vi "CODMn通讯.vi"() -> ()   [LabVIEW 2016, in "斯坦道CODMn新电路板.lvlib"]
uses:
  <vilib>/NI/Modbus Library/API/Wrapper/Create TCP Slave.vi
  <vilib>/Utility/config.llb/Write Key (String).vi
  <vilib>/Plasmionique/MB Master/MB_Master/MB_Master.lvclass
  <vilib>/NI/Modbus Library/API/Slave/Modbus Slave.lvclass
  <vilib>/Utility/config.llb/NI_LVConfig.lvlib
  <vilib>/Plasmionique/MB Master/MB Master.lvlib
  <vilib>/NI/Modbus Library/API/Wrapper/API Main.lvlib
panel:
  out "控制命令 2":u16[](array[numeric]) format="%xH"
  out "状态告警区":T1 {"工作状态" items=["空闲"=0, "水样测试"=1, "标样核查"=2, "零点核查"=3, "跨度核查"=4, "空白测试"=5, "平行样测试"=6, "加标回收"=7, "空白校准"=8, "标样校准"=9, "初始化（清洗）"=10, "调试"=22, "填充管路"=30, "清洗管路"=31, "清洗反应杯"=32]; "告警代码" items=["无告警", "缺试剂告警", "缺水样告警", "缺蒸馏水告警", "缺标液告警", "仪表漏液告警", "标定异常告警", "超量程告警", "加热异常", "低试剂预警", "超上限告警", "超下限告警", "仪表内部其他异常", "滴定异常告警", "电极异常告警", "量程切换告警", "参数设置告警", "PH电极电位异常", "电导率电极异常", "浊度光度异常", "溶解氧电极异常", "溶解氧光强异常", "温度异常告警", "PH异常告警", "溶解氧异常告警", "电导率异常告警", "浊度异常告警", "叶绿素异常告警", "藻密度异常告警", "蓝绿藻异常告警", "ORP异常告警", "氨氮异常告警", "清洁刷异常告警", "SD卡异常告警", "蓝牙异常告警", "Wifi异常告警", "流程异常告警"]; "故障代码" items=["无故障", "电机故障", "温度故障", "通讯故障", "滴定故障"]}
  out "测量数据区":T2 {"单位" items=["ug/L", "mg/L", "ppm", "mg/m3", "cm", "ppb", "ug/m3", "%", "nmol/mol", "umol/mol", "MPN/L", "MPN/100ml", "ng/m3", "NTU", "无量纲", "ms/cm", "us/cm", "℃", "mV", "万个/L"]}
  out "状态告警区":u16[](array[numeric])
  out "测量数据区":u16[](array[numeric])
  out "序列号":string
  out "status":bool
  out "关键参数区":T3
  in  "读关键参数区":bool
  in  "读状态告警区":bool
  in  "读测量数据区":bool
  in  "站号":u16(ring) items=["CODMn"=21, "氨氮"=3]
  in  "停止":bool
  in  "启动":bool
  in  "控制命令":u16(ring) items=["启动测量"=1, "标样核查"=2, "零点核查"=3, "跨度核查"=4, "空白测试"=5, "平行样测试"=6, "加标回收"=7, "空白校准"=8, "标样校准"=9, "初始化（清洗）"=10, "停止测试"=11, "仪器重启"=12, "校时"=13, "模式设置"=14, "测量间隔设置"=15]
  in  "控制命令参数":u16[](array[numeric]) format="%04xH"
  in  "VISA Resource":refnum<visa-resource-name>
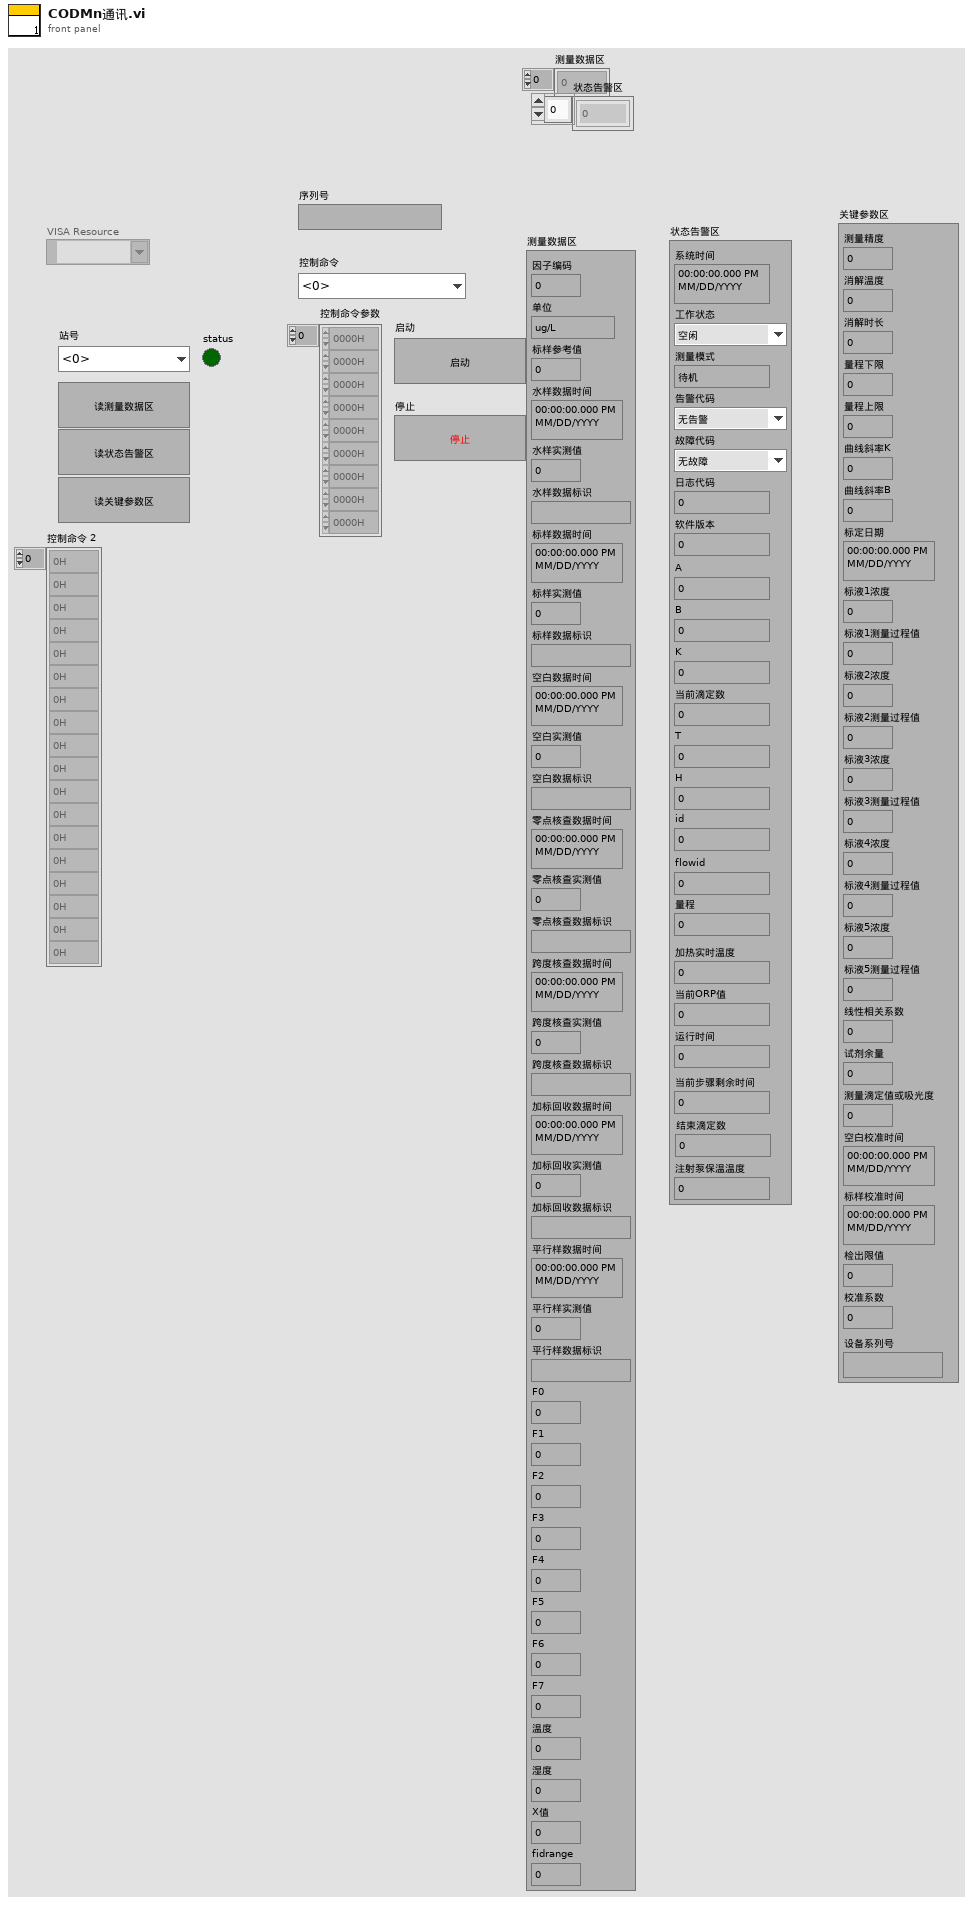
[diagram p1: front panel]
types:
  T1 = cluster{"系统时间":timestamp, "工作状态":u16, "测量模式":enum16{"待机", "连续模式", "周期模式", "定点模式", "受控模式", "手动模式"}, "告警代码":u16, "故障代码":u16, "日志代码":u16, "软件版本":u16, "A":sgl, "B":sgl, "K":sgl, "当前滴定数":sgl, "T":sgl, "H":sgl, "id":u16, "flowid":u16, "量程":u16, "加热实时温度":sgl, "当前ORP值":sgl, "运行时间":sgl, "当前步骤剩余时间":sgl, "结束滴定数":sgl, "注射泵保温温度":sgl}
  T2 = cluster{"因子编码":u32, "单位":u16, "标样参考值":sgl, "水样数据时间":timestamp, "水样实测值":sgl, "水样数据标识":string, "标样数据时间":timestamp, "标样实测值":sgl, "标样数据标识":string, "空白数据时间":timestamp, "空白实测值":sgl, "空白数据标识":string, "零点核查数据时间":timestamp, "零点核查实测值":sgl, "零点核查数据标识":string, "跨度核查数据时间":timestamp, "跨度核查实测值":sgl, "跨度核查数据标识":string, "加标回收数据时间":timestamp, "加标回收实测值":sgl, "加标回收数据标识":string, "平行样数据时间":timestamp, "平行样实测值":sgl, "平行样数据标识":string, "F0":sgl, "F1":sgl, "F2":sgl, "F3":sgl, "F4":sgl, "F5":sgl, "F6":sgl, "F7":sgl, "温度":sgl, "湿度":sgl, "X值":sgl, "fidrange":sgl}
  T3 = cluster{"测量精度":u16, "消解温度":u16, "消解时长":u16, "量程下限":sgl, "量程上限":sgl, "曲线斜率K":sgl, "曲线斜率B":sgl, "标定日期":timestamp, "标液1浓度":sgl, "标液1测量过程值":sgl, "标液2浓度":sgl, "标液2测量过程值":sgl, "标液3浓度":sgl, "标液3测量过程值":sgl, "标液4浓度":sgl, "标液4测量过程值":sgl, "标液5浓度":sgl, "标液5测量过程值":sgl, "线性相关系数":sgl, "试剂余量":u32, "测量滴定值或吸光度":sgl, "空白校准时间":timestamp, "标样校准时间":timestamp, "检出限值":sgl, "校准系数":sgl, "设备系列号":string}
  T4 = cluster{"测量模式":enum16{"水样测量", "标样核查", "零点核查", "跨度核查", "空白测试", "加标回收", "平行样", "校零", "校标"}}
  T5 = typedef "NI_LVConfig.lvlib/Config Data RefNum.ctl" = refnum<k1>
  T6 = cluster{"站号":u16, "量程切换":enum32{"H", "L", "AUTO"}, "控制命令":u16, "模式设置":enum16{"待机", "连续模式", "周期模式", "定点模式", "受控模式", "手动模式"}, "测量间隔":u16}
  T7 = enum16{"水样测量", "标样核查", "零点核查", "跨度核查", "空白测试", "加标回收", "平行样", "校零", "校标"}
  T8 = enum8{"Enabled", "Disabled", "Disabled and Grayed Out"}
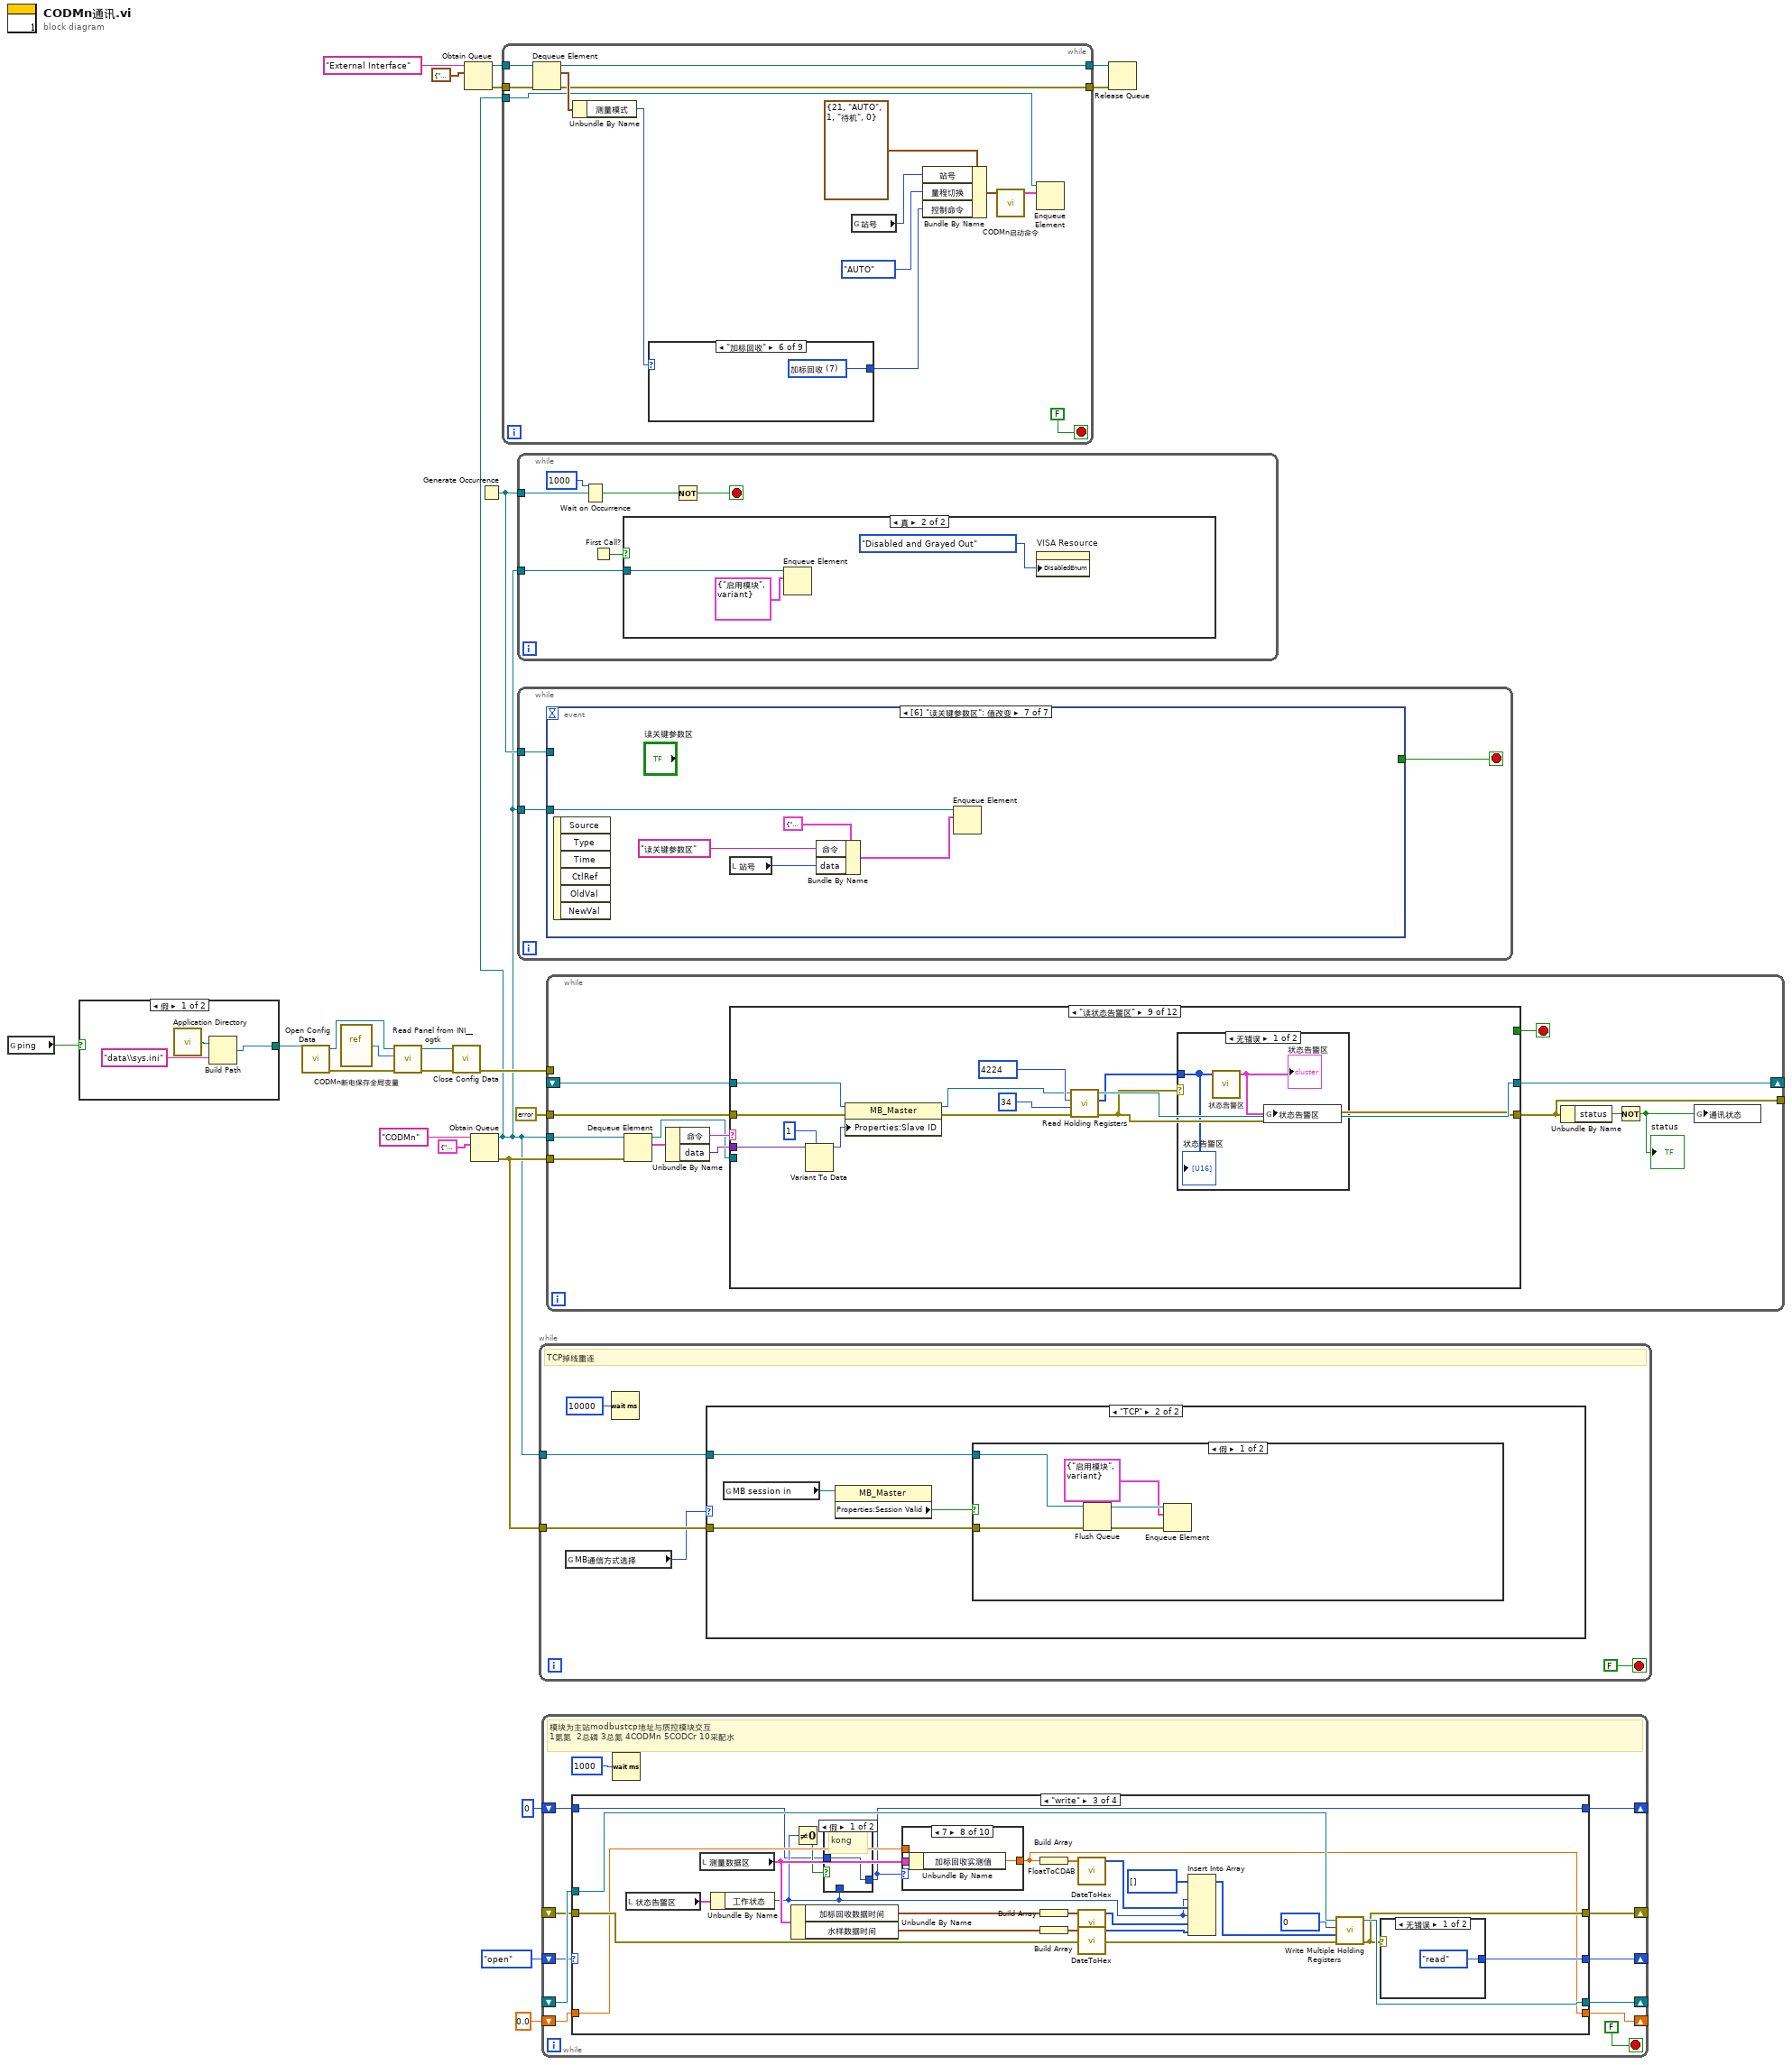
[diagram p0: block diagram]
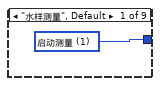
[diagram p2: hidden frame]
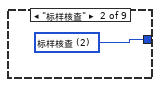
[diagram p3: hidden frame]
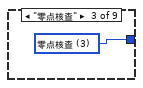
[diagram p4: hidden frame]
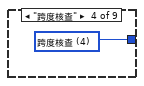
[diagram p5: hidden frame]
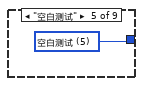
[diagram p6: hidden frame]
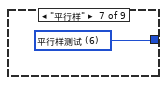
[diagram p7: hidden frame]
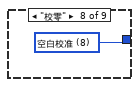
[diagram p8: hidden frame]
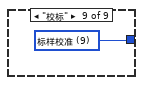
[diagram p9: hidden frame]
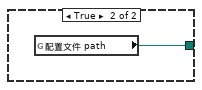
[diagram p10: hidden frame]
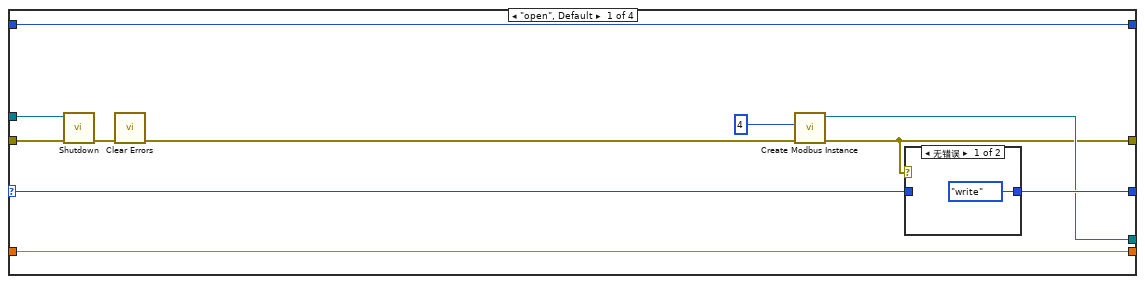
[diagram p13: hidden frame]
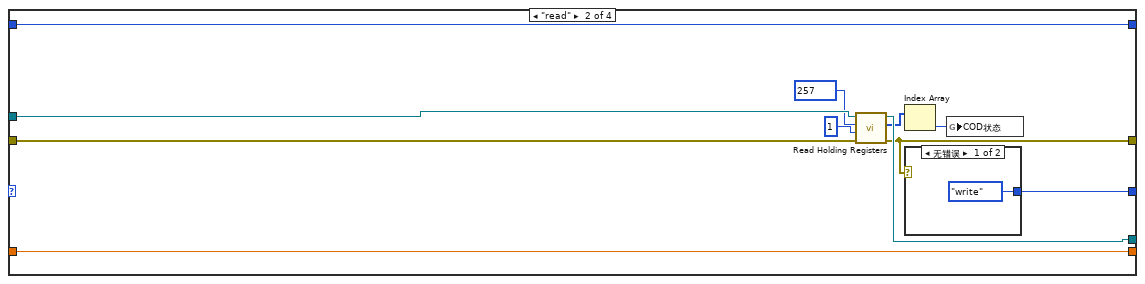
[diagram p15: hidden frame]
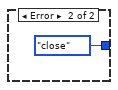
[diagram p16: hidden frame]
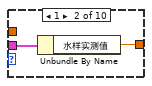
[diagram p19: hidden frame]
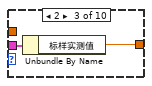
[diagram p20: hidden frame]
diagram:
  n1 = global read "VARCODMn全局变量.vi" "ping"() -> (w11:bool)
  n2 = case shown="假" w11 {
    tunnel: [w24 w27] -> w10
    frame False {
      n3 = call <vilib>:"Application Directory.vi"() -> ("Application Directory"=w26:path)
      n4 = Build Path(base path=w26, name or relative path="data\\sys.ini" ("名称或相对路径")) -> (appended path=w24:path)
    }
    frame True {
      n5 = global read "VARCODMn全局变量.vi" "配置文件 path"() -> (w27:path)
    }
  }
  n6 = call <vilib>:"Open Config Data.vi"("configuration file path"=w10) -> ("error out"=w18:errorcluster, "refnum"=w15:T5)  [unwired: 8 in, 1 out]
  n7 = vi-ref "CODMn断电保存全局变量.vi"() -> (w16:refnum<vi>)
  n8 = call <userlib>:"Read Panel from INI__ogtk.vi"("error in (no error)"=w18, "VI ref"=w16, "refnum"=w15) -> ("error out"=w19:errorcluster, "refnum out"=w17:T5)  [unwired: 7 in]
  n9 = call <vilib>:"Close Config Data.vi"("error in (no error)"=w19, "refnum"=w17) -> ("error out"=w14:errorcluster)  [unwired: 8 in, 1 out]
  n10 = Obtain Queue(name (unnamed)="External Interface" ("名称（未命名）"), element data type=T4 {"测量模式"=enum."水样测量"} ("元素")) -> (queue out=w7:refnum<queue>, error out=w6:errorcluster)  [unwired: 3 in, 1 out]
  n11 = Obtain Queue(name (unnamed)="CODMn" ("名称（未命名）"), element data type=cluster{"命令":string, "data":variant} {"命令"="", "data"=variant}) -> (queue out=w5:refnum<queue>, error out=w12:errorcluster)  [unwired: 3 in, 1 out]
  n12 = Generate Occurrence() -> (w20:refnum<k4>)
  n13 = while {
    tunnel: w7 -> [w41]
    tunnel: w6 -> [w40]
    tunnel: w5 -> [w32]
    tunnel: [w31] -> w4
    tunnel: [w30] -> w3
    stop <- FALSE stop-if-true
    n14 = Dequeue Element(queue=w41, error in (no error)=w40) -> (queue out=w31:refnum<queue>, element=w35:T4, error out=w30:errorcluster)  [unwired: 1 in, 1 out]
    n15 = Unbundle By Name(w35) -> ("测量模式"=w34:T7)
    n16 = case shown="\"加标回收\"" w34 {
      tunnel: [w42 w43 w44 w45 w46 w47 w48 w49 w50] -> w33
      frame "水样测量", Default {
        w42 = u16 1 items=["启动测量"=1, "标样核查"=2, "零点核查"=3, "跨度核查"=4, "空白测试"=5, "平行样测试"=6, "加标回收"=7, "空白校准"=8, "标样校准"=9, "初始化（清洗）"=10, "停止测试"=11, "仪器重启"=12, "校时"=13, "模式设置"=14, "测量间隔设置"=15, "调试"=22, "填充管路"=30, "清洗管路"=31, "清洗反应杯"=32] ("控制命令")
      }
      frame "标样核查" {
        w43 = u16 2 items=["启动测量"=1, "标样核查"=2, "零点核查"=3, "跨度核查"=4, "空白测试"=5, "平行样测试"=6, "加标回收"=7, "空白校准"=8, "标样校准"=9, "初始化（清洗）"=10, "停止测试"=11, "仪器重启"=12, "校时"=13, "模式设置"=14, "测量间隔设置"=15, "调试"=22, "填充管路"=30, "清洗管路"=31, "清洗反应杯"=32] ("控制命令")
      }
      frame "零点核查" {
        w44 = u16 3 items=["启动测量"=1, "标样核查"=2, "零点核查"=3, "跨度核查"=4, "空白测试"=5, "平行样测试"=6, "加标回收"=7, "空白校准"=8, "标样校准"=9, "初始化（清洗）"=10, "停止测试"=11, "仪器重启"=12, "校时"=13, "模式设置"=14, "测量间隔设置"=15, "调试"=22, "填充管路"=30, "清洗管路"=31, "清洗反应杯"=32] ("控制命令")
      }
      frame "跨度核查" {
        w45 = u16 4 items=["启动测量"=1, "标样核查"=2, "零点核查"=3, "跨度核查"=4, "空白测试"=5, "平行样测试"=6, "加标回收"=7, "空白校准"=8, "标样校准"=9, "初始化（清洗）"=10, "停止测试"=11, "仪器重启"=12, "校时"=13, "模式设置"=14, "测量间隔设置"=15, "调试"=22, "填充管路"=30, "清洗管路"=31, "清洗反应杯"=32] ("控制命令")
      }
      frame "空白测试" {
        w46 = u16 5 items=["启动测量"=1, "标样核查"=2, "零点核查"=3, "跨度核查"=4, "空白测试"=5, "平行样测试"=6, "加标回收"=7, "空白校准"=8, "标样校准"=9, "初始化（清洗）"=10, "停止测试"=11, "仪器重启"=12, "校时"=13, "模式设置"=14, "测量间隔设置"=15, "调试"=22, "填充管路"=30, "清洗管路"=31, "清洗反应杯"=32] ("控制命令")
      }
      frame "加标回收" {
        w47 = u16 7 items=["启动测量"=1, "标样核查"=2, "零点核查"=3, "跨度核查"=4, "空白测试"=5, "平行样测试"=6, "加标回收"=7, "空白校准"=8, "标样校准"=9, "初始化（清洗）"=10, "停止测试"=11, "仪器重启"=12, "校时"=13, "模式设置"=14, "测量间隔设置"=15, "调试"=22, "填充管路"=30, "清洗管路"=31, "清洗反应杯"=32] ("控制命令")
      }
      frame "平行样" {
        w48 = u16 6 items=["启动测量"=1, "标样核查"=2, "零点核查"=3, "跨度核查"=4, "空白测试"=5, "平行样测试"=6, "加标回收"=7, "空白校准"=8, "标样校准"=9, "初始化（清洗）"=10, "停止测试"=11, "仪器重启"=12, "校时"=13, "模式设置"=14, "测量间隔设置"=15, "调试"=22, "填充管路"=30, "清洗管路"=31, "清洗反应杯"=32] ("控制命令")
      }
      frame "校零" {
        w49 = u16 8 items=["启动测量"=1, "标样核查"=2, "零点核查"=3, "跨度核查"=4, "空白测试"=5, "平行样测试"=6, "加标回收"=7, "空白校准"=8, "标样校准"=9, "初始化（清洗）"=10, "停止测试"=11, "仪器重启"=12, "校时"=13, "模式设置"=14, "测量间隔设置"=15, "调试"=22, "填充管路"=30, "清洗管路"=31, "清洗反应杯"=32] ("控制命令")
      }
      frame "校标" {
        w50 = u16 9 items=["启动测量"=1, "标样核查"=2, "零点核查"=3, "跨度核查"=4, "空白测试"=5, "平行样测试"=6, "加标回收"=7, "空白校准"=8, "标样校准"=9, "初始化（清洗）"=10, "停止测试"=11, "仪器重启"=12, "校时"=13, "模式设置"=14, "测量间隔设置"=15, "调试"=22, "填充管路"=30, "清洗管路"=31, "清洗反应杯"=32] ("控制命令")
      }
    }
    n17 = global read "CODMn断电保存全局变量.vi" "站号"() -> (w36:u16)
    n18 = Bundle By Name(cluster=T6 {"站号"=21, "量程切换"=enum."AUTO", "控制命令"=1, "模式设置"=enum."待机", "测量间隔"=0} ("参数"), "站号"=w36, "量程切换"=enum32{"H", "L", "AUTO"}."AUTO", "控制命令"=w33) -> (w37:T6)
    n19 = call "CODMn启动命令.vi"("参数"=w37) -> ("启动命令"=w39:cluster{"命令":string, "data":variant})  [unwired: 10 in]
    n20 = Enqueue Element(queue=w32, element=w39) -> ()  [unwired: 2 in, 3 out]
  }
  n21 = while {
    tunnel: w20 -> [w56]
    tunnel: w5 -> [w52]
    stop <- w53 stop-if-true
    n22 = Wait on Occurrence(2:w56, 3:1000 ("毫秒超时(-1)")) -> (0:w54:bool)  [unwired: 1 in]
    n23 = First Call?() -> (First Call?: T/F=w51:bool)
    n24 = case shown="真" w51 {
      tunnel: w52 -> [_ w58]
      frame False {
      }
      frame True {
        n25 = Enqueue Element(queue=w58, element=cluster{"命令":string, "data":variant} {"命令"="启用模块", "data"=variant} ("元素")) -> ()  [unwired: 2 in, 3 out]
        n26 = property on="VISA Resource" class="VISAName"("DisabledEnum"=T8."Disabled and Grayed Out" ("禁用")) -> ()  [unwired: 2 in, 2 out]
      }
    }
    n27 = Not(x=w54) -> (.not. x?=w53:bool)
  }
  n28 = while {
    tunnel: w5 -> [w62]
    tunnel: w20 -> [w60]
    stop <- w61 stop-if-true
    n29 = event shown="[6] \"读关键参数区\": 值改变" {
      selector: _ -> [_ _ _ _ _ _ _]
      dyn-events: _ -> [_ _ _ _ _ _ _]
      timeout: _ -> [_ _ _ _ _ _ _]
      tunnel: w62 -> [_ _ w83 w90 w96 w101 w106]
      tunnel: [_ _ _ "停止" _ _ _] -> w61
      tunnel: w60 -> [_ _ _ w87 _ _ _]
      event Timeout {
        n30 = event-data() -> ()  [unwired: 1 in, 3 out]
      }
      event "VISA Resource": Value Change {
        n31 = event-data() -> ()  [unwired: 1 in, 6 out]
        n32 = call <vilib>:"Application Directory.vi"() -> ("Application Directory"=w65:path)
        n33 = Build Path(base path=w65, name or relative path="data\\set.ini" ("名称或相对路径")) -> (appended path=w66:path)
        n34 = call <vilib>:"Open Config Data.vi"("configuration file path"=w66) -> ("error out"=w72:errorcluster, "refnum"=w71:T5)  [unwired: 8 in, 1 out]
        n35 = call-poly <vilib>:"Write Key.vi"("section"="CODMn", "error in (no error)"=w72, "value"="VISA Resource", "key"="串口", "refnum"=w71) -> ("error out"=w68:errorcluster, "refnum out"=w64:T5)  [unwired: 4 in, 1 out]
        n36 = call <vilib>:"Close Config Data.vi"("error in (no error)"=w68, "refnum"=w64) -> ()  [unwired: 8 in, 2 out]
      }
      event "启动": Value Change {
        n37 = event-data() -> ()  [unwired: 1 in, 6 out]
        n38 = case shown="默认" "控制命令" {
          tunnel: "控制命令参数" -> [w85 w86]
          tunnel: [w84 w86] -> w73
          frame Default {
            n39 = call "HexToWord.vi"("数组"=w85) -> ("WORD"=w84:u16[])  [unwired: 10 in]
          }
          frame 13 {
          }
        }
        n40 = Swap Bytes(anything="控制命令") -> (byte swapped=w76:u16)
        n41 = call "控制命令区.vi"("控制命令参数"=w73, "控制命令"=w76) -> ("控制命令"=w79:u16[])  [unwired: 9 in]
        n42 = local read "站号"() -> (w78:u16)
        n43 = Bundle("站号"=w78, "控制命令"=w79) -> (w77:cluster{"站号":u16, "控制命令":u16[]})  [unwired: 1 in]
        n44 = Bundle By Name(cluster=cluster{"命令":string, "data":variant} {"命令"="", "data"=variant} ("元素"), "命令"="启动", "data"=w77) -> (w81:cluster{"命令":string, "data":variant})
        n45 = Enqueue Element(queue=w83, element=w81) -> ()  [unwired: 2 in, 3 out]
      }
      event "停止": Value Change {
        n46 = event-data() -> ()  [unwired: 1 in, 6 out]
        n47 = Set Occurrence(w87) -> ()
        n48 = Flush Queue(queue=w90) -> (queue out=w89:refnum<queue>)  [unwired: 1 in, 2 out]
        n49 = Enqueue Element(queue=w89, element=cluster{"命令":string, "data":variant} {"命令"="shutdown", "data"=variant} ("元素")) -> ()  [unwired: 2 in, 3 out]
      }
      event "读测量数据区": Value Change {
        n50 = event-data() -> ()  [unwired: 1 in, 6 out]
        n51 = Bundle By Name(cluster=cluster{"命令":string, "data":variant} {"命令"="", "data"=variant} ("元素"), "命令"="读测量数据区", "data"="站号") -> (w94:cluster{"命令":string, "data":variant})
        n52 = Enqueue Element(queue=w96, element=w94) -> ()  [unwired: 2 in, 3 out]
      }
      event "读状态告警区": Value Change {
        n53 = event-data() -> ()  [unwired: 1 in, 6 out]
        n54 = local read "站号"() -> (w97:u16)
        n55 = Bundle By Name(cluster=cluster{"命令":string, "data":variant} {"命令"="", "data"=variant} ("元素"), "命令"="读状态告警区", "data"=w97) -> (w99:cluster{"命令":string, "data":variant})
        n56 = Enqueue Element(queue=w101, element=w99) -> ()  [unwired: 2 in, 3 out]
      }
      event "读关键参数区": Value Change {
        n57 = event-data() -> ()  [unwired: 1 in, 6 out]
        n58 = local read "站号"() -> (w102:u16)
        n59 = Bundle By Name(cluster=cluster{"命令":string, "data":variant} {"命令"="", "data"=variant} ("元素"), "命令"="读关键参数区", "data"=w102) -> (w104:cluster{"命令":string, "data":variant})
        n60 = Enqueue Element(queue=w106, element=w104) -> ()  [unwired: 2 in, 3 out]
      }
    }
  }
  n61 = while "While循环" {
    tunnel: w5 -> [w109]
    tunnel: w12 -> [w108]
    stop <- FALSE stop-if-true
    # "TCP掉线重连"
    n62 = global read "CODMn断电保存全局变量.vi" "MB通信方式选择"() -> (w107:enum16{"串口", "TCP"})
    n63 = Wait (ms)(milliseconds to wait=u32 10000 ("等待时间（毫秒）")) -> ()  [unwired: 1 out]
    n64 = case shown="\"TCP\"" w107 {
      tunnel: w109 -> [_ w114]
      tunnel: w108 -> [_ w113]
      frame "串口", Default {
      }
      frame "TCP" {
        n65 = global read "VARCODMn全局变量.vi" "MB session in"() -> (w112:refnum<class "MB_Master.lvclass">)
        n66 = property class="MB_Master"(reference=w112) -> ("Properties:Session Valid"=w115:bool)  [unwired: 1 in, 2 out]
        n67 = case shown="假" w115 {
          tunnel: w114 -> [w118 _]
          tunnel: w113 -> [w117 _]
          frame False {
            n68 = Flush Queue(queue=w118, error in (no error)=w117) -> (queue out=w120:refnum<queue>, error out=w119:errorcluster)  [unwired: 1 out]
            n69 = Enqueue Element(queue=w120, element=cluster{"命令":string, "data":variant} {"命令"="启用模块", "data"=variant} ("元素"), error in (no error)=w119) -> ()  [unwired: 1 in, 3 out]
          }
          frame True {
          }
        }
      }
    }
  }
  n70 = while {
    shift-right: [w130] -> _
    shift-left: _ -> [w132]
    shift-right: [w129] -> _
    shift-left: _ -> [w131]
    shift-right: [w126] -> _
    shift-left: enum16{"open", "read", "write", "close"}."open" -> [w127]
    shift-right: [w124] -> _
    shift-left: sgl 0.0 ("标样实测值") -> [w123]
    shift-right: [w122] -> _
    shift-left: u16 0 ("工作状态") -> [w121]
    stop <- FALSE stop-if-true
    # "模块为主站modbustcp地址与质控模块交互\n1氨氮  2总磷 3总氮 4CODMn 5CODCr 10采配水"
    n71 = case shown="\"write\"" w127 {
      selector: w127 -> [w143 _ _ _]
      tunnel: w132 -> [w137 w155 w181 w210]
      tunnel: w131 -> [w136 w153 w180 w209]
      tunnel: [w140 w154 w178 w210] -> w130
      tunnel: [w139 w152 w177 w212] -> w129
      tunnel: [w142 w156 w182 enum16{"open", "read", "write", "close"}."open"] -> w126
      tunnel: [w134 w147 w172 w207] -> w124
      tunnel: w123 -> [w134 w147 w173 w207]
      tunnel: [w133 w146 w160 w206] -> w122
      tunnel: w121 -> [w133 w146 w159 w206]
      frame "open", Default {
        n72 = call-dynamic "Shutdown.vi"("error in"=w136, "Modbus slave in"=w137) -> ("error out"=w135:errorcluster)  [unwired: 9 in]
        n73 = call <vilib>:"Clear Errors.vi"("error in (no error)"=w135) -> ("error out"=w138:errorcluster)  [unwired: 5 in, 1 out]
        n74 = call-poly <vilib>:"Create Modbus Instance.vi"("error in"=w138, "port (502)"=u16 4) -> ("error out"=w139:errorcluster, "TCP slave instance"=w140:refnum<class "Modbus Slave.lvclass">)  [unwired: 8 in]
        n75 = case shown="无错误" w139 {
          tunnel: w143 -> [_ w145]
          tunnel: [enum16{"open", "read", "write", "close"}."write" w145] -> w142
          frame No Error {
          }
          frame Error {
          }
        }
      }
      frame "read" {
        n76 = call-dynamic <vilib>:"Read Holding Registers.vi"("error in"=w153, "number of inputs"=u16 1, "starting address"=u16 257, "Modbus slave in"=w155) -> ("error out"=w152:errorcluster, "register values"=w149:u16[], "Modbus slave out"=w154:refnum<class "Modbus Slave.lvclass">)  [unwired: 5 in]
        n77 = Index Array(array=w149) -> (element=w148:u16)  [unwired: 1 in]
        n78 = case shown="无错误" w152 {
          tunnel: [enum16{"open", "read", "write", "close"}."write" enum16{"open", "read", "write", "close"}."close"] -> w156
          frame No Error {
          }
          frame Error {
          }
        }
        n79 = global write "VARCODMn全局变量.vi" "COD状态"(w148) -> ()
      }
      frame "write" {
        n80 = local read "状态告警区"() -> (w174:T1)
        n81 = local read "测量数据区"() -> (w169:T2)
        n82 = Unbundle By Name(w174) -> ("工作状态"=w161:u16)
        n83 = Unbundle By Name(w169) -> ("加标回收数据时间"=w168:timestamp, "水样数据时间"=w165:timestamp)
        n84 = Not Equal To 0?(x=w161) -> (x != 0?=w162:bool)
        n85 = case shown="假" w162 {
          tunnel: w161 -> [_ w184]
          tunnel: [w183 w184] -> w160
          tunnel: w159 -> [w183 _]
          frame False {
            # "kong"
          }
          frame True {
            # "..."
          }
        }
        n86 = case shown="7" w160 {
          tunnel: [w185 w187 w189 w191 w193 w195 w197 w199 w201 w203] -> w172
          tunnel: w173 -> [w185 _ _ _ _ _ _ _ _ _]
          tunnel: w169 -> [_ w186 w188 w190 w192 w194 w196 w198 w200 w202]
          frame 0, Default {
          }
          frame 1 {
            n87 = Unbundle By Name(w186) -> ("水样实测值"=w187:sgl)
          }
          frame 2 {
            n88 = Unbundle By Name(w188) -> ("标样实测值"=w189:sgl)
          }
          frame 3 {
            n89 = Unbundle By Name(w190) -> ("零点核查实测值"=w191:sgl)
          }
          frame 4 {
            n90 = Unbundle By Name(w192) -> ("跨度核查实测值"=w193:sgl)
          }
          frame 5 {
            n91 = Unbundle By Name(w194) -> ("空白实测值"=w195:sgl)
          }
          frame 6 {
            n92 = Unbundle By Name(w196) -> ("平行样实测值"=w197:sgl)
          }
          frame 7 {
            n93 = Unbundle By Name(w198) -> ("加标回收实测值"=w199:sgl)
          }
          frame 8 {
            n94 = Unbundle By Name(w200) -> ("空白实测值"=w201:sgl)
          }
          frame 9 {
            n95 = Unbundle By Name(w202) -> ("标样实测值"=w203:sgl)
          }
        }
        n96 = Build Array(w172) -> (w171:sgl[])
        n97 = Build Array(w168) -> (w167:timestamp[])
        n98 = Build Array(w165) -> (w164:timestamp[])
        n99 = call "FloatToCDAB.vi"("浮点数"=w171) -> ("CDAB整形输出"=w170:u16[])  [unwired: 10 in]
        n100 = call "DateToHex.vi"("DATE"=w167) -> ("数组"=w166:u16[])  [unwired: 10 in]
        n101 = call "DateToHex.vi"("DATE"=w164) -> ("数组"=w163:u16[])  [unwired: 10 in]
        n102 = Insert Into Array(array=u16[] [] ("values"), new element #1=w161, new element #2=w170, new element #3=w161, new element #4=w166, new element #5=w163) -> (w175:u16[])  [unwired: 1 in]
        n103 = call-dynamic "Write Multiple Holding Registers.vi"("error in"=w180, "registers to write"=w175, "starting address"=u16 0, "Modbus slave in"=w181) -> ("error out"=w177:errorcluster, "Modbus slave out"=w178:refnum<class "Modbus Slave.lvclass">)  [unwired: 6 in]
        n104 = case shown="无错误" w177 {
          tunnel: [enum16{"open", "read", "write", "close"}."read" enum16{"open", "read", "write", "close"}."close"] -> w182
          frame No Error {
          }
          frame Error {
          }
        }
      }
      frame "close" {
        n105 = call-dynamic "Shutdown.vi"("error in"=w209, "Modbus slave in"=w210) -> ("error out"=w208:errorcluster)  [unwired: 9 in]
        n106 = call <vilib>:"Clear Errors.vi"("error in (no error)"=w208) -> ("error out"=w212:errorcluster)  [unwired: 5 in, 1 out]
      }
    }
    n107 = Wait (ms)(milliseconds to wait=u32 1000 ("等待时间（毫秒）")) -> ()  [unwired: 1 out]
  }
  n108 = while {
    tunnel: w5 -> [w225]
    tunnel: w12 -> [w224]
    shift-right: [w222] -> _
    shift-left: _ -> [w221]
    tunnel: errorcluster {"status"=FALSE, "code"=0, "source"=""} ("error out") -> [w220]
    tunnel: [w215] -> _
    tunnel: w14 -> [_]
    stop <- w223 stop-if-true
    n109 = Dequeue Element(queue=w225, error in (no error)=w224) -> (queue out=w216:refnum<queue>, element=w218:cluster{"命令":string, "data":variant})  [unwired: 1 in, 2 out]
    n110 = Unbundle By Name(w218) -> ("命令"=w219:string, "data"=w217:variant)
    n111 = case shown="\"读状态告警区\"" w219 {
      tunnel: w217 -> [_ _ _ w244 w255 w272 w284 w293 w303 w319 w334 _]
      tunnel: w216 -> [_ _ _ _ _ _ _ _ _ _ _ w347]
      tunnel: [_ _ _ _ _ _ _ _ _ _ _ TRUE] -> w223
      tunnel: [w226 w229 w231 w247 w258 w274 w286 w298 w312 w326 w341 w343] -> w222
      tunnel: [w227 w228 w232 w246 w257 w273 w285 w287 w301 w315 w342 w344] -> w215
      tunnel: w221 -> [w226 _ w231 w243 w254 w271 w283 w292 w306 w322 w337 w343]
      tunnel: w220 -> [w227 _ w234 w240 w251 w268 w280 w290 w307 w323 w338 w345]
      frame Default {
      }
      frame "启用模块" {
        n112 = call "MB_api.vi"("STEP"=enum16{"open", "read", "write", "close"}."open") -> ("error out"=w228:errorcluster, "MB session out"=w229:refnum<class "MB_Master.lvclass">)  [unwired: 8 in, 1 out]
        n113 = global write "VARCODMn全局变量.vi" "MB session in"(w229) -> ()
      }
      frame "停用模块" {
        n114 = call-dynamic "Close Session.vi"("error in (no error)"=w234, "MB session in"=w231) -> ("error out"=w233:errorcluster)  [unwired: 9 in]
        n115 = call <vilib>:"Clear Errors.vi"("error in (no error)"=w233) -> ("error out"=w232:errorcluster)  [unwired: 5 in, 1 out]
      }
      frame "启动" {
        n116 = Variant To Data(type=cluster{"站号":u16, "控制命令":u16[]} {"站号"=0, "控制命令"=[]} ("输出簇"), Variant=w244) -> (data=w238:cluster{"站号":u16, "控制命令":u16[]})  [unwired: 1 in, 1 out]
        n117 = Unbundle By Name(w238) -> ("站号"=w237:u16, "控制命令"=w235:u16[])
        n118 = property class="MB_Master"(reference=w243, error in=w240, "Properties:Slave ID"=w237) -> (reference out=w242:refnum<class "MB_Master.lvclass">, error out=w241:errorcluster)
        n119 = Index Array(array=w235) -> (element=w236:u16)  [unwired: 1 in]
        n120 = global write "VARCODMn全局变量.vi" "控制命令"(w236) -> ()
        n121 = call <vilib>:"Write Multiple Registers.vi"("error in (no error)"=w241, "values"=w235, "starting address"=u16 4608, "MB session in"=w242) -> ("error out"=w246:errorcluster, "MB session out"=w247:refnum<class "MB_Master.lvclass">)  [unwired: 6 in]
      }
      frame "盲样测试" {
        n122 = Variant To Data(type=0, Variant=w255) -> (data=w248:i32)  [unwired: 1 in, 1 out]
        n123 = property class="MB_Master"(reference=w254, error in=w251, "Properties:Slave ID"=w248) -> (reference out=w253:refnum<class "MB_Master.lvclass">, error out=w252:errorcluster)
        n124 = case shown="默认" w248 {
          tunnel: [u16[] [] ("values") u16[] [33539, 0] ("values") u16[] [23555, 0] ("values")] -> w250
          frame Default {
          }
          frame 1 {
            # "总磷盲样测试命令"
          }
          frame 3 {
            # "氨氮盲样测试"
          }
        }
        n125 = call <vilib>:"Write Multiple Registers.vi"("error in (no error)"=w252, "values"=w250, "starting address"=u16 24592, "MB session in"=w253) -> ("error out"=w257:errorcluster, "MB session out"=w258:refnum<class "MB_Master.lvclass">)  [unwired: 6 in]
      }
      frame "debug" {
        n126 = Variant To Data(type=cluster{"站号":u16, "控制命令":u16[]} {"站号"=0, "控制命令"=[]} ("输出簇"), Variant=w272) -> (data=w266:cluster{"站号":u16, "控制命令":u16[]})  [unwired: 1 in, 1 out]
        n127 = Unbundle By Name(w266) -> ("站号"=w265:u16, "控制命令"=w263:u16[])
        "控制命令 2" <- w263
        n128 = property class="MB_Master"(reference=w271, error in=w268, "Properties:Slave ID"=w265) -> (reference out=w270:refnum<class "MB_Master.lvclass">, error out=w269:errorcluster)
        n129 = Index Array(array=w263) -> (element=w264:u16)  [unwired: 1 in]
        n130 = global write "VARCODMn全局变量.vi" "控制命令"(w264) -> ()
        n131 = call <vilib>:"Write Multiple Registers.vi"("error in (no error)"=w269, "values"=w263, "starting address"=u16 24594, "MB session in"=w270) -> ("error out"=w273:errorcluster, "MB session out"=w274:refnum<class "MB_Master.lvclass">)  [unwired: 6 in]
      }
      frame "单步控制" {
        n132 = Variant To Data(type=cluster{"站号":u16, "控制命令":u16[]} {"站号"=0, "控制命令"=[]} ("输出簇"), Variant=w284) -> (data=w278:cluster{"站号":u16, "控制命令":u16[]})  [unwired: 1 in, 1 out]
        n133 = Unbundle By Name(w278) -> ("站号"=w277:u16, "控制命令"=w276:u16[])
        n134 = property class="MB_Master"(reference=w283, error in=w280, "Properties:Slave ID"=w277) -> (reference out=w282:refnum<class "MB_Master.lvclass">, error out=w281:errorcluster)
        n135 = call <vilib>:"Write Multiple Registers.vi"("error in (no error)"=w281, "values"=w276, "starting address"=u16 24610, "MB session in"=w282) -> ("error out"=w285:errorcluster, "MB session out"=w286:refnum<class "MB_Master.lvclass">)  [unwired: 6 in]
      }
      frame "读测量数据区" {
        n136 = Variant To Data(type=u8 1 ("Slave ID"), Variant=w293) -> (data=w294:u8)  [unwired: 1 in, 1 out]
        n137 = property class="MB_Master"(reference=w292, error in=w290, "Properties:Slave ID"=w294) -> (reference out=w291:refnum<class "MB_Master.lvclass">, error out=w289:errorcluster)
        n138 = call <vilib>:"Read Holding Registers.vi"("error in (no error)"=w289, "quantity"=u16 105, "starting address"=u16 4096, "MB session in"=w291) -> ("error out"=w287:errorcluster, "Registers"=w288:u16[], "MB session out"=w298:refnum<class "MB_Master.lvclass">)  [unwired: 5 in]
        n139 = case shown="无错误" w287 {
          tunnel: w288 -> [w300 _]
          frame No Error {
            n140 = call "测量数据区.vi"("数组"=w300) -> ("测量数据区"=w299:T2)  [unwired: 10 in]
            "测量数据区" <- w299
            n141 = global write "VARCODMn全局变量.vi" "测量数据区"(w299) -> ()
            "测量数据区" <- w300
          }
          frame Error {
          }
        }
      }
      frame "读状态告警区" {
        n142 = Variant To Data(type=u8 1 ("Slave ID"), Variant=w303) -> (data=w308:u8)  [unwired: 1 in, 1 out]
        n143 = property class="MB_Master"(reference=w306, error in=w307, "Properties:Slave ID"=w308) -> (reference out=w305:refnum<class "MB_Master.lvclass">, error out=w304:errorcluster)
        n144 = call <vilib>:"Read Holding Registers.vi"("error in (no error)"=w304, "quantity"=u16 34, "starting address"=u16 4224, "MB session in"=w305) -> ("error out"=w301:errorcluster, "Registers"=w302:u16[], "MB session out"=w312:refnum<class "MB_Master.lvclass">)  [unwired: 5 in]
        n145 = case shown="无错误" w301 {
          tunnel: w302 -> [w314 _]
          frame No Error {
            n146 = call "状态告警区.vi"("数组"=w314) -> ("状态告警区"=w313:T1)  [unwired: 10 in]
            "状态告警区" <- w313
            n147 = global write "VARCODMn全局变量.vi" "状态告警区"(w313) -> ()
            "状态告警区" <- w314
          }
          frame Error {
          }
        }
      }
      frame "读关键参数区" {
        n148 = Variant To Data(type=u8 1 ("Slave ID"), Variant=w319) -> (data=w317:u8)  [unwired: 1 in, 1 out]
        n149 = property class="MB_Master"(reference=w322, error in=w323, "Properties:Slave ID"=w317) -> (reference out=w321:refnum<class "MB_Master.lvclass">, error out=w320:errorcluster)
        n150 = call <vilib>:"Read Holding Registers.vi"("error in (no error)"=w320, "quantity"=u16 19, "starting address"=u16 4256, "MB session in"=w321) -> ("error out"=w315:errorcluster, "Registers"=w316:u16[], "MB session out"=w326:refnum<class "MB_Master.lvclass">)  [unwired: 5 in]
        n151 = case shown="无错误" w315 {
          tunnel: w316 -> [w328 _]
          frame No Error {
            n152 = call "关键参数区.vi"("数组"=w328) -> ("关键参数区"=w327:T3)  [unwired: 10 in]
            "关键参数区" <- w327
            n153 = global write "VARCODMn全局变量.vi" "关键参数区"(w327) -> ()
          }
          frame Error {
          }
        }
      }
      frame "读序列号" {
        n154 = Variant To Data(type=u8 1 ("Slave ID"), Variant=w334) -> (data=w332:u8)  [unwired: 1 in, 1 out]
        n155 = property class="MB_Master"(reference=w337, error in=w338, "Properties:Slave ID"=w332) -> (reference out=w336:refnum<class "MB_Master.lvclass">, error out=w335:errorcluster)
        n156 = call <vilib>:"Read Holding Registers.vi"("error in (no error)"=w335, "quantity"=u16 6, "starting address"=u16 4, "MB session in"=w336) -> ("error out"=w342:errorcluster, "Registers"=w331:u16[], "MB session out"=w341:refnum<class "MB_Master.lvclass">)  [unwired: 5 in]
        n157 = call "HexToString.vi"("数组"=w331) -> ("STRING"=w330:string[])  [unwired: 10 in]
        n158 = Index Array(array=w330) -> (element=w329:string)  [unwired: 1 in]
        "序列号" <- w329
        n159 = global write "VARCODMn全局变量.vi" "序列号"(w329) -> ()
      }
      frame "shutdown" {
        n160 = call-dynamic "Close Session.vi"("error in (no error)"=w345, "MB session in"=w343) -> ("error out"=w344:errorcluster)  [unwired: 9 in]
        n161 = Flush Queue(queue=w347) -> (queue out=w346:refnum<queue>)  [unwired: 1 in, 2 out]
        n162 = Release Queue(queue=w346) -> ()  [unwired: 2 in, 3 out]
      }
    }
    n163 = Unbundle By Name(w215) -> ("status"=w214:bool)
    n164 = Not(x=w214) -> (.not. x?=w213:bool)
    "status" <- w213
    n165 = global write "VARCODMn全局变量.vi" "通讯状态"(w213) -> ()
  }
  n166 = Release Queue(queue=w4, error in (no error)=w3) -> ()  [unwired: 1 in, 3 out]
